vi "Numberpad.vi"(8 "Error In":errorcluster) -> (0 "Error Out":errorcluster, 3 "Value":dbl)   [LabVIEW 2017]
panel:
  in  "Cluster":T1
  out "Number":string
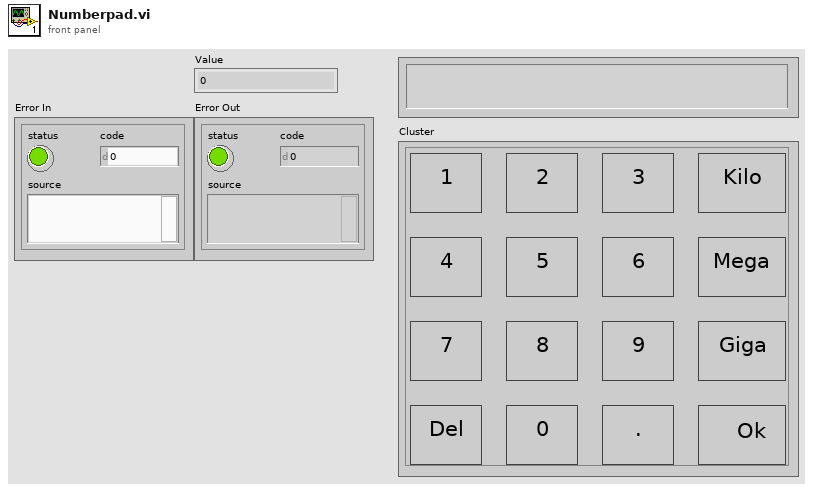
[diagram p1: front panel]
types:
  T1 = cluster{"Button 1":bool, "Button 2":bool, "Button 3":bool, "Button 4":bool, "Button 5":bool, "Button 6":bool, "Button 7":bool, "Button 8":bool, "Button 9":bool, "Button 10":bool, "Button K":bool, "Button M":bool, "Button G":bool, "Button Decimal":bool, "Delete":bool, "Button Ok":bool}
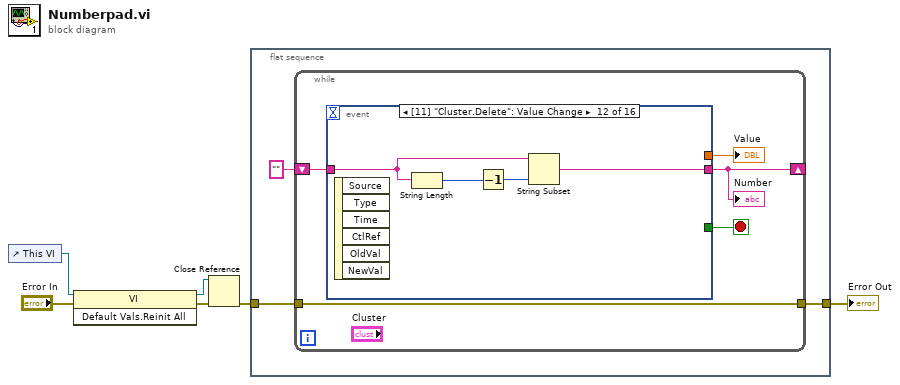
[diagram p0: block diagram]
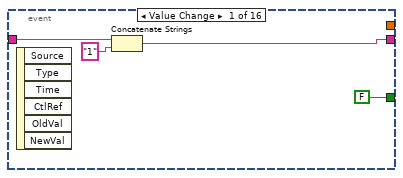
[diagram p2: hidden frame]
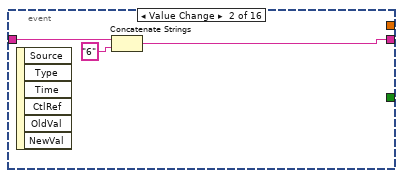
[diagram p3: hidden frame]
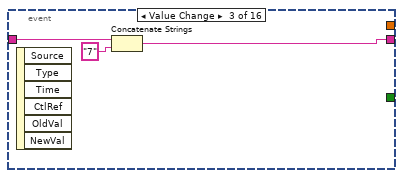
[diagram p4: hidden frame]
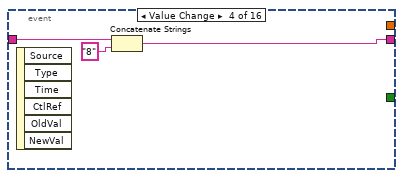
[diagram p5: hidden frame]
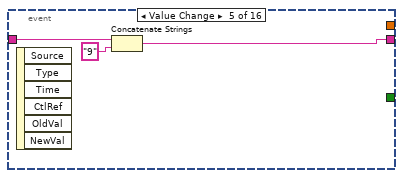
[diagram p6: hidden frame]
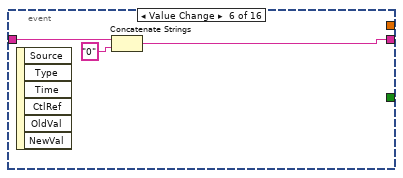
[diagram p7: hidden frame]
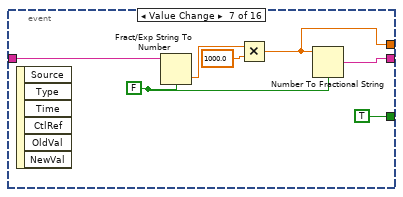
[diagram p8: hidden frame]
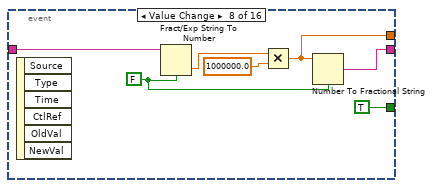
[diagram p9: hidden frame]
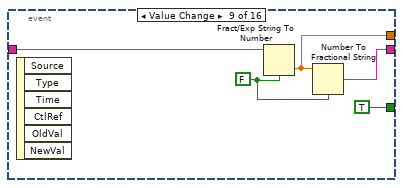
[diagram p10: hidden frame]
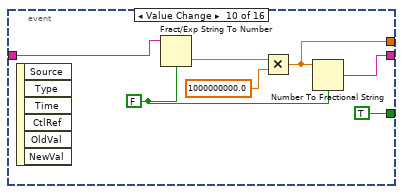
[diagram p11: hidden frame]
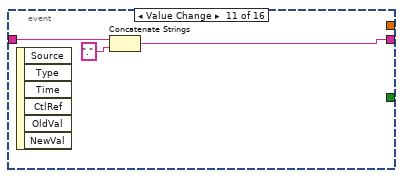
[diagram p12: hidden frame]
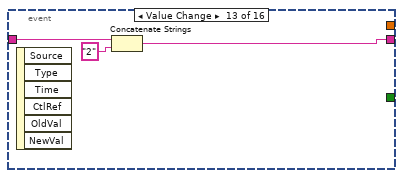
[diagram p13: hidden frame]
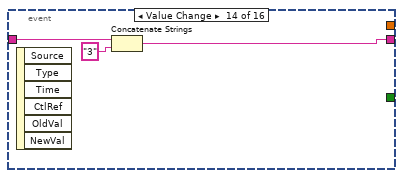
[diagram p14: hidden frame]
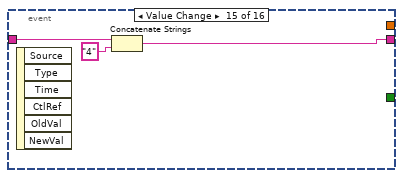
[diagram p15: hidden frame]
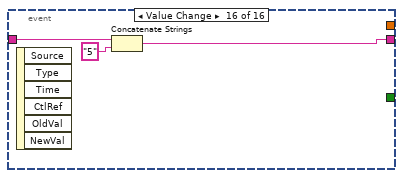
[diagram p16: hidden frame]
diagram:
  n1 = control-ref of="This VI"() -> (w6:refnum<vi>)
  n2 = invoke class="VI" method="Default Vals.Reinit All"(reference=w6, error in="Error In") -> (reference out=w4:refnum<vi>, error out=w5:errorcluster)  [unwired: 1 in, 1 out]
  n3 = Close Reference(reference=w4, error in (no error)=w5) -> (error out=w3:errorcluster)
  n4 = flat-sequence {
    tunnel: [w9] -> w1
    tunnel: w3 -> [w7]
    frame #0 {
      n5 = while {
        shift-right: [w12] -> _
        shift-left: "" -> [w14]
        tunnel: w7 -> [w10]
        tunnel: [w10] -> w9
        stop <- w13 stop-if-true
        n6 = event shown="[11] \"Cluster.Delete\": Value Change" {
          selector: _ -> [_ _ _ _ _ _ _ _ _ _ _ _ _ _ _ _]
          dyn-events: _ -> [_ _ _ _ _ _ _ _ _ _ _ _ _ _ _ _]
          timeout: _ -> [_ _ _ _ _ _ _ _ _ _ _ _ _ _ _ _]
          tunnel: w14 -> [w16 w20 w23 w26 w28 w32 w40 w44 w51 w56 w62 w66 w67 w71 w74 w76]
          tunnel: [w18 w21 w24 w27 w30 w33 w36 w43 w49 w53 w61 w63 w69 w72 w75 w78] -> w12
          tunnel: [FALSE _ _ _ _ _ TRUE TRUE TRUE TRUE _ _ _ _ _ _] -> w13
          tunnel: [_ _ _ _ _ _ w37 w42 w48 w55 _ _ _ _ _ _] -> w11
          event "Cluster.Button 1": Value Change {
            n7 = event-data() -> ()  [unwired: 1 in, 6 out]
            n8 = Concatenate Strings(w16, "1" ("string")) -> (w18:string)
          }
          event "Cluster.Button 6": Value Change {
            n9 = event-data() -> ()  [unwired: 1 in, 6 out]
            n10 = Concatenate Strings(w20, "6" ("string")) -> (w21:string)
          }
          event "Cluster.Button 7": Value Change {
            n11 = event-data() -> ()  [unwired: 1 in, 6 out]
            n12 = Concatenate Strings(w23, "7" ("string")) -> (w24:string)
          }
          event "Cluster.Button 8": Value Change {
            n13 = event-data() -> ()  [unwired: 1 in, 6 out]
            n14 = Concatenate Strings(w26, "8" ("string")) -> (w27:string)
          }
          event "Cluster.Button 9": Value Change {
            n15 = event-data() -> ()  [unwired: 1 in, 6 out]
            n16 = Concatenate Strings(w28, "9" ("string")) -> (w30:string)
          }
          event "Cluster.Button 10": Value Change {
            n17 = event-data() -> ()  [unwired: 1 in, 6 out]
            n18 = Concatenate Strings(w32, "0" ("string")) -> (w33:string)
          }
          event "Cluster.Button K": Value Change {
            w35 = FALSE ("use system decimal point (T)")
            n19 = event-data() -> ()  [unwired: 1 in, 6 out]
            n20 = Fract/Exp String To Number(use system decimal point (T)=w35, string=w40) -> (number=w39:dbl)  [unwired: 2 in, 1 out]
            n21 = Multiply(x=w39, y=1000.0) -> (x*y=w37:dbl)
            n22 = Number To Fractional String(use system decimal point (T)=w35, number=w37) -> (F-format string=w36:string)  [unwired: 2 in]
          }
          event "Cluster.Button M": Value Change {
            w45 = FALSE ("use system decimal point (T)")
            n23 = event-data() -> ()  [unwired: 1 in, 6 out]
            n24 = Fract/Exp String To Number(use system decimal point (T)=w45, string=w44) -> (number=w47:dbl)  [unwired: 2 in, 1 out]
            n25 = Multiply(x=w47, y=1000000.0) -> (x*y=w42:dbl)
            n26 = Number To Fractional String(use system decimal point (T)=w45, number=w42) -> (F-format string=w43:string)  [unwired: 2 in]
          }
          event "Cluster.Button Ok": Value Change {
            w52 = FALSE ("use system decimal point (T)")
            n27 = event-data() -> ()  [unwired: 1 in, 6 out]
            n28 = Fract/Exp String To Number(use system decimal point (T)=w52, string=w51) -> (number=w48:dbl)  [unwired: 2 in, 1 out]
            n29 = Number To Fractional String(use system decimal point (T)=w52, number=w48) -> (F-format string=w49:string)  [unwired: 2 in]
          }
          event "Cluster.Button G": Value Change {
            w57 = FALSE ("use system decimal point (T)")
            n30 = event-data() -> ()  [unwired: 1 in, 6 out]
            n31 = Fract/Exp String To Number(use system decimal point (T)=w57, string=w56) -> (number=w59:dbl)  [unwired: 2 in, 1 out]
            n32 = Multiply(x=w59, y=1000000000.0) -> (x*y=w55:dbl)
            n33 = Number To Fractional String(use system decimal point (T)=w57, number=w55) -> (F-format string=w53:string)  [unwired: 2 in]
          }
          event "Cluster.Button Decimal": Value Change {
            n34 = event-data() -> ()  [unwired: 1 in, 6 out]
            n35 = Concatenate Strings(w62, "." ("string")) -> (w61:string)
          }
          event "Cluster.Delete": Value Change {
            n36 = event-data() -> ()  [unwired: 1 in, 6 out]
            n37 = String Length(string=w66) -> (length=w64:i32)
            n38 = Decrement(x=w64) -> (x-1=w65:i32)
            n39 = String Subset(string=w66, length (rest)=w65) -> (substring=w63:string)  [unwired: 1 in]
          }
          event "Cluster.Button 2": Value Change {
            n40 = event-data() -> ()  [unwired: 1 in, 6 out]
            n41 = Concatenate Strings(w67, "2" ("string")) -> (w69:string)
          }
          event "Cluster.Button 3": Value Change {
            n42 = event-data() -> ()  [unwired: 1 in, 6 out]
            n43 = Concatenate Strings(w71, "3" ("string")) -> (w72:string)
          }
          event "Cluster.Button 4": Value Change {
            n44 = event-data() -> ()  [unwired: 1 in, 6 out]
            n45 = Concatenate Strings(w74, "4" ("string")) -> (w75:string)
          }
          event "Cluster.Button 5": Value Change {
            n46 = event-data() -> ()  [unwired: 1 in, 6 out]
            n47 = Concatenate Strings(w76, "5" ("string")) -> (w78:string)
          }
        }
        "Number" <- w12
        "Value" <- w11
      }
    }
  }
  "Error Out" <- w1
